vi "home position.vi"(8 "error in (no error)":errorcluster, 10 "yhome":i16, 11 "xhome":i16) -> (0 "error out":errorcluster)   [LabVIEW 2015, in "SCANalone4x64.lvlib"]
doc: "__declspec(dllimport) void __stdcall home_position(short xhome, short yhome);"
uses:
  <userlib>/SCANalone4x64/SCANalone4x64.lvlib
  <userlib>/SCANalone4x64/SCANalone4x64.dll
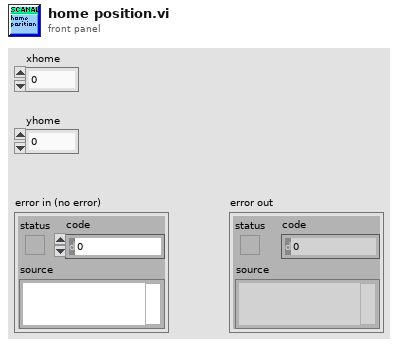
[diagram p1: front panel]
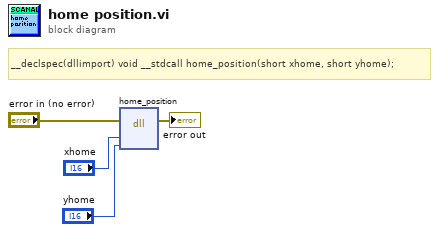
[diagram p0: block diagram]
diagram:
  # "__declspec(dllimport) void __stdcall home_position(short xhome, short yhome);"
  n1 = dll-call lib="C:/Program Files/National Instruments/LabVIEW 2015/user.lib/SCANalone4x64/SCANalone4x64.*" fn="home_position"(error in="error in (no error)", "xhome"="xhome", "yhome"="yhome") -> (error out=→"error out":errorcluster)  [unwired: 5 in, 1 out]
